vi "Find Next Position of H.vi"(0 "Current Position of H":cdb, 1 "Movement Direction":string) -> (2 "Next Position of H":cdb)   [LabVIEW 2020, in "AoC 2022.lvlib"]
uses:
  AoC 2022.lvlib
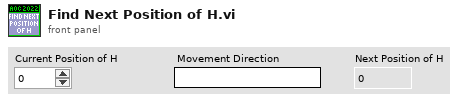
[diagram p1: front panel]
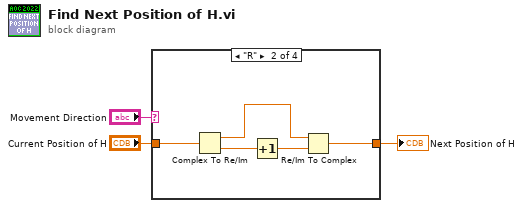
[diagram p0: block diagram]
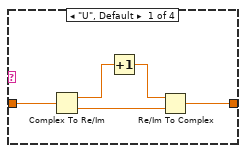
[diagram p2: hidden frame]
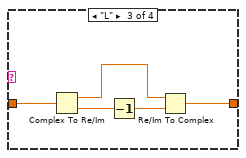
[diagram p3: hidden frame]
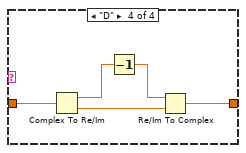
[diagram p4: hidden frame]
diagram:
  n1 = case shown="\"R\"" "Movement Direction" {
    tunnel: "Current Position of H" -> [w8 w13 w18 w23]
    tunnel: [w7 w12 w17 w22] -> w3
    frame "U", Default {
      n2 = Complex To Re/Im(x + iy=w8) -> (x=w5:dbl, y=w6:dbl)
      n3 = Increment(x=w5) -> (x+1=w4:dbl)
      n4 = Re/Im To Complex(1:w6, 2:w4) -> (0:w7:cdb)
    }
    frame "R" {
      n5 = Complex To Re/Im(x + iy=w13) -> (x=w9:dbl, y=w11:dbl)
      n6 = Increment(x=w11) -> (x+1=w10:dbl)
      n7 = Re/Im To Complex(1:w10, 2:w9) -> (0:w12:cdb)
    }
    frame "L" {
      n8 = Complex To Re/Im(x + iy=w18) -> (x=w14:dbl, y=w16:dbl)
      n9 = Decrement(x=w16) -> (x-1=w15:dbl)
      n10 = Re/Im To Complex(1:w15, 2:w14) -> (0:w17:cdb)
    }
    frame "D" {
      n11 = Complex To Re/Im(x + iy=w23) -> (x=w20:dbl, y=w21:dbl)
      n12 = Decrement(x=w20) -> (x-1=w19:dbl)
      n13 = Re/Im To Complex(1:w21, 2:w19) -> (0:w22:cdb)
    }
  }
  "Next Position of H" <- w3
